vi "DataFlowComplete_Parse.vi"(8 "error in (no error)":errorcluster, 11 "body":variant) -> (0 "error out":errorcluster, 3 "group":string)   [LabVIEW 2017, in "DataFlow.lvlib"]
doc: "Converts the data set from the previous process in the Dataflow Script from variant data to its original cluster format."
uses:
  <vilib>/addons/InsightCM/Devices/Shared/Common/DataFlow/DataFlow.lvlib
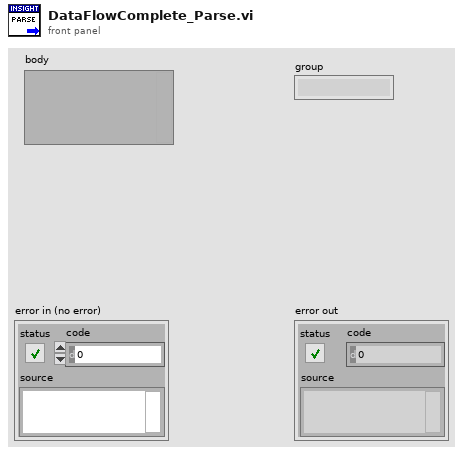
[diagram p1: front panel]
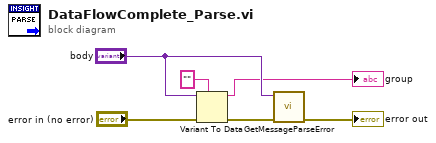
[diagram p0: block diagram]
diagram:
  n1 = Variant To Data(error in="error in (no error)", type="", Variant="body") -> (data=→"group":string, error out=w6:errorcluster)
  n2 = call <vilib>:"GetMessageParseError.vi"("error in (no error)"=w6, "body"="body") -> ("error out"=→"error out":errorcluster)  [unwired: 7 in, 2 out]
